vi "Close Seq File Ref.vi"(8 "error in (no error)":errorcluster, 9 "options":i32, 10 "Seq File Ref":refnum<k7>, 11 "Engine Ref":refnum<k7>) -> (0 "error out":errorcluster)   [LabVIEW 2014, in "teststand-api.lvlib" / "teststand-api.lvclass"]
uses:
  teststand-api.lvclass
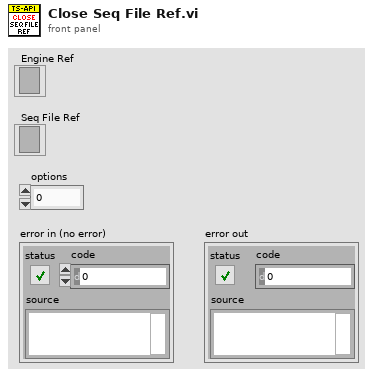
[diagram p1: front panel]
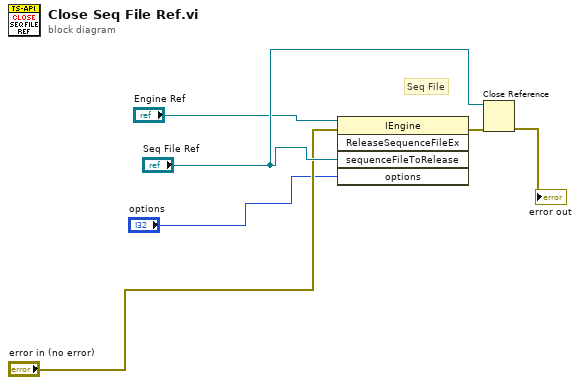
[diagram p0: block diagram]
diagram:
  # "Seq File"
  n1 = invoke class="IEngine" method="ReleaseSequenceFileEx"(reference="Engine Ref", error in="error in (no error)", "sequenceFileToRelease"="Seq File Ref", "options"="options") -> (error out=w4:errorcluster)  [unwired: 1 in, 4 out]
  n2 = Close Reference(reference="Seq File Ref", error in (no error)=w4) -> (error out=→"error out":errorcluster)
